vi "Histogram Main.vi"() -> ()   [LabVIEW 2012]
uses:
  Consumer Message.ctl
panel:
  out "波形图表":dbl[](graph)
  in  "快照":bool
  out "直方图":cluster{"histogram":dbl[], "x axis":dbl[]}(graph)
  out "消费者关闭？":bool
  in  "停止":bool
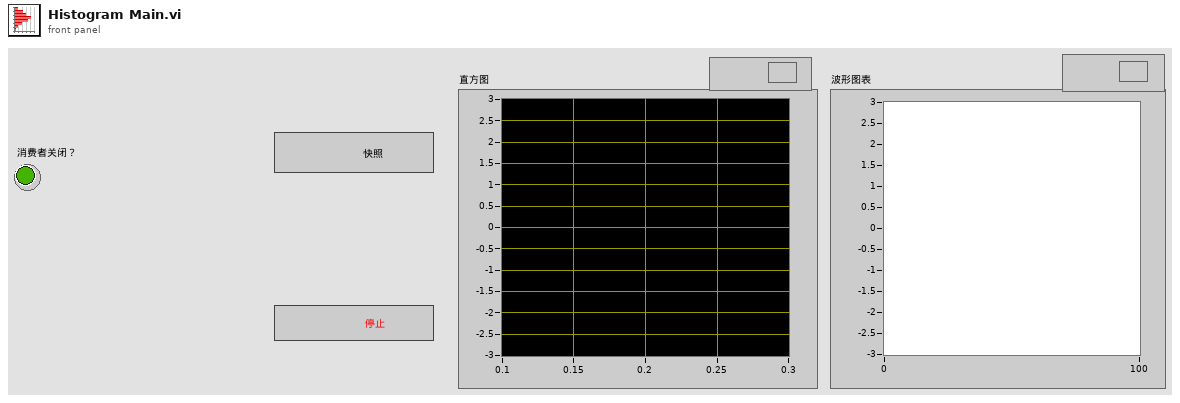
[diagram p1: front panel]
types:
  T1 = typedef "Consumer Message.ctl" = cluster{"消费者状态":string, "布尔数据":bool, "数值数据":i32, "信号":dbl[], "错误":cluster{"状态":bool, "代码":i32, "源":string}}
  T2 = enum32{"invalid app kind", "Development System", "Run Time System", "Student Edition", "Embedded LabVIEW", "Evaluation", "Custom"}
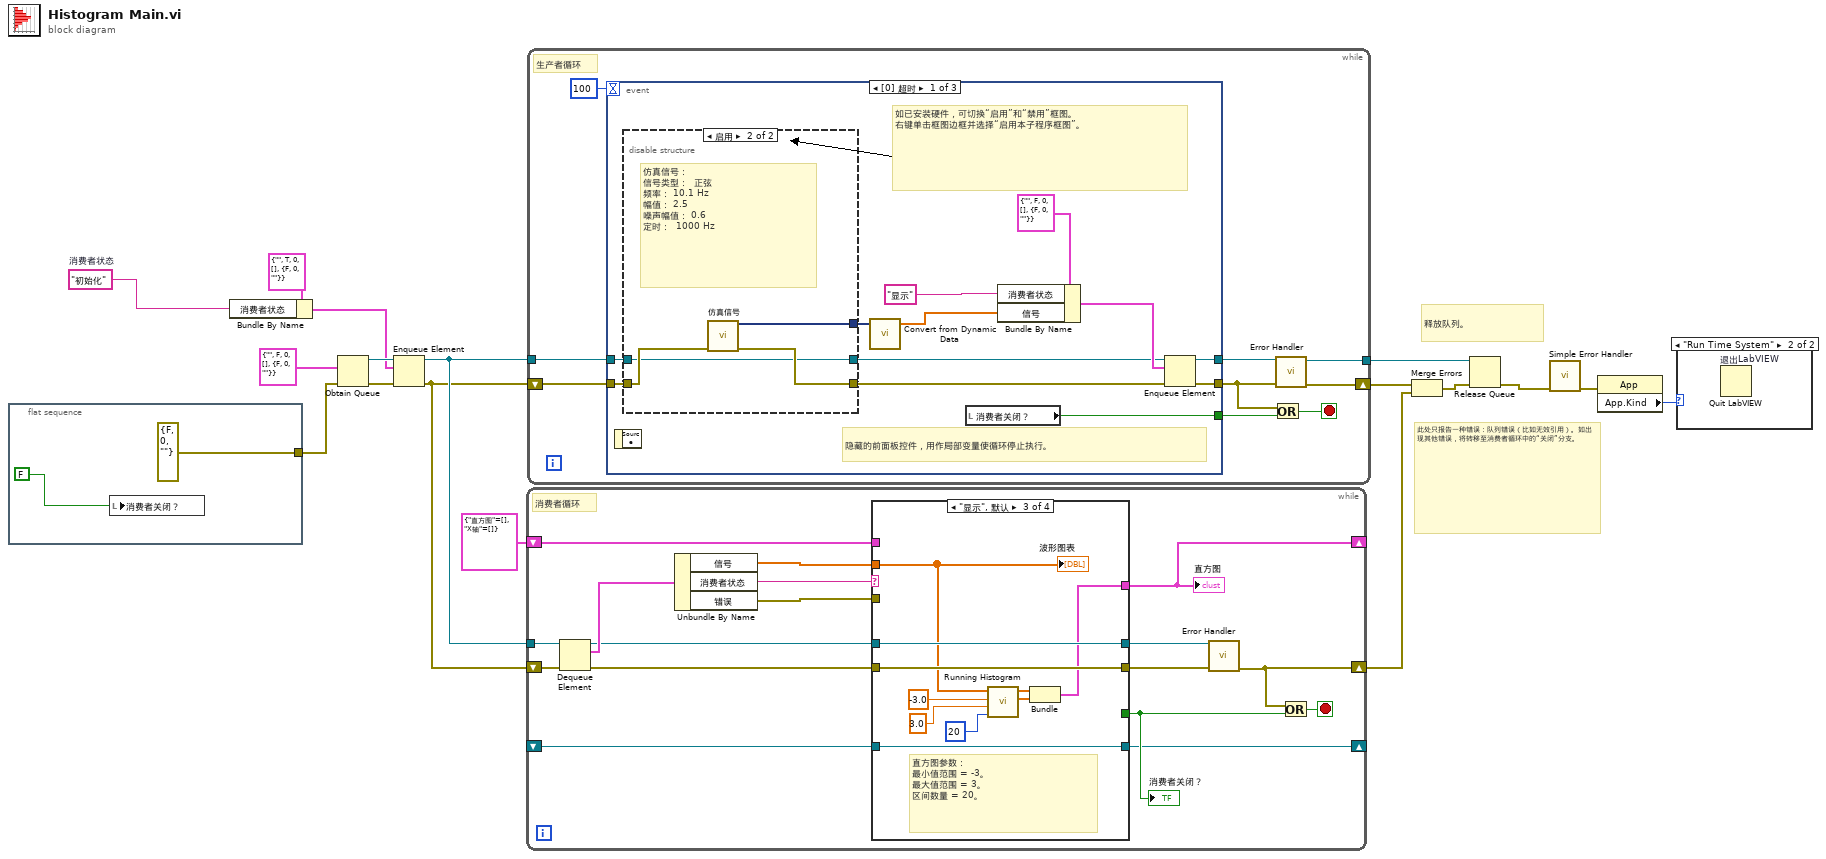
[diagram p0: block diagram]
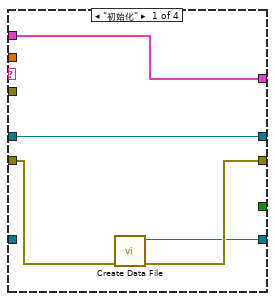
[diagram p3: hidden frame]
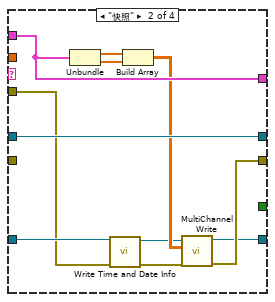
[diagram p4: hidden frame]
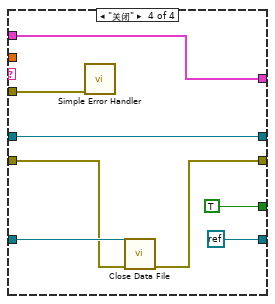
[diagram p5: hidden frame]
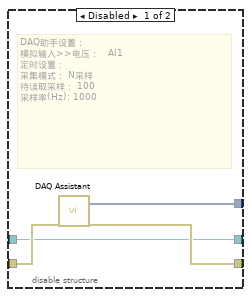
[diagram p6: hidden frame]
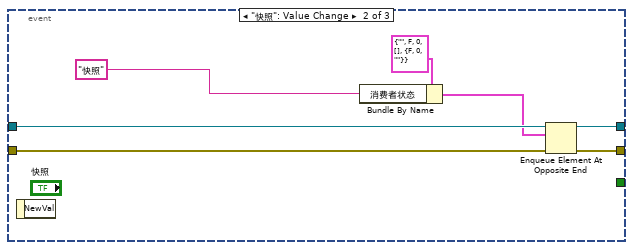
[diagram p7: hidden frame]
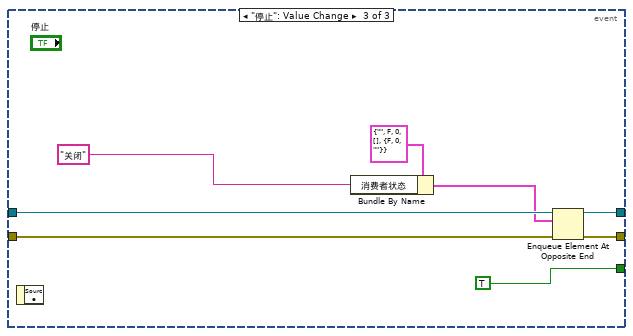
[diagram p8: hidden frame]
diagram:
  w10 = "初始化"  # 消费者状态
  # "释放队列。"
  # "此处只报告一种错误：队列错误（比如无效引用）。如出现其他错误，将转移至消费者循环中的“关闭”分支。"
  n1 = flat-sequence {
    tunnel: [cluster{"状态":bool, "代码":i32, "源":string} {"状态"=FALSE, "代码"=0, "源"=""} ("错误输入（无错误）")] -> w13
    frame #0 {
      n2 = local write "消费者关闭？"(FALSE ("停止循环（局部）")) -> ()
    }
  }
  n3 = Bundle By Name ("按名称捆绑")(cluster=T1 {"消费者状态"="", "布尔数据"=TRUE, "数值数据"=0, "信号"=[], "错误"={"状态"=FALSE, "代码"=0, "源"=""}} ("消费者消息"), "消费者状态"=w10) -> (w11:T1)
  n4 = Obtain Queue ("获取队列引用")(element data type=T1 {"消费者状态"="", "布尔数据"=FALSE, "数值数据"=0, "信号"=[], "错误"={"状态"=FALSE, "代码"=0, "源"=""}}, error in (no error)=w13) -> (queue out=w15:refnum<queue>, error out=w17:errorcluster)  [unwired: 3 in, 1 out]
  n5 = Enqueue Element ("元素入队列")(queue=w15, element=w11, error in (no error)=w17) -> (queue out=w14:refnum<queue>, error out=w4:errorcluster)  [unwired: 1 in, 1 out]
  n6 = while {
    tunnel: w14 -> [w36]
    shift-right: [w27] -> w8
    shift-left: w4 -> [w35]
    shift-right: [w20] -> _
    shift-left: cluster{"直方图":dbl[], "X轴":dbl[]} {"直方图"=[], "X轴"=[]} -> [w24]
    shift-right: [w21] -> _
    shift-left: _ -> [w22]
    stop <- w28 stop-if-true
    # "消费者循环"
    n7 = Dequeue Element ("元素出队列")(queue=w36, error in (no error)=w35) -> (queue out=w26:refnum<queue>, element=w34:T1, error out=w25:errorcluster)  [unwired: 1 in, 1 out]
    n8 = Unbundle By Name ("按名称解除捆绑")(w34) -> ("信号"=w23:dbl[], "消费者状态"=w33:string, "错误"=w30:cluster{"状态":bool, "代码":i32, "源":string})
    n9 = case shown="\"显示\", 默认" w33 {
      tunnel: [_ _ _ TRUE] -> w29
      tunnel: w25 -> [w39 _ w61 w65]
      tunnel: [w38 w48 w61 w64] -> w32
      tunnel: w26 -> [w41 w52 w62 w68]
      tunnel: [w41 w52 w62 w68] -> w31
      tunnel: w30 -> [_ w42 _ w69]
      tunnel: [w40 w50 w58 w67] -> w20
      tunnel: w24 -> [w40 w50 _ w67]
      tunnel: w23 -> [_ _ w56 _]
      tunnel: w22 -> [_ w43 w57 w66]
      tunnel: [w37 w47 w57 refnum<k0> refnum ("非法引用句柄常量")] -> w21
      frame "初始化" {
        n10 = call "Create Data File.vi"("错误输入"=w39) -> ("错误输出"=w38:cluster{"状态":bool, "代码":i32, "源":string}, "文件引用句柄"=w37:refnum<file>)  [unwired: 9 in]
      }
      frame "快照" {
        n11 = Unbundle ("解除捆绑")(w50) -> ("直方图"=w46:dbl[], "X轴"=w51:dbl[])
        n12 = call "Write Time and Date Info.vi"("错误输入"=w42, "文件引用句柄输入"=w43) -> ("错误输出"=w44:cluster{"状态":bool, "代码":i32, "源":string}, "文件引用句柄输出"=w45:refnum<file>)  [unwired: 6 in]
        n13 = Build Array ("创建数组")(w46, w51) -> (w49:dbl[][])
        n14 = call "MultiChannel Write.vi"("错误输入"=w44, "数据至记录"=w49, "文件引用句柄输入"=w45) -> ("错误输出"=w48:cluster{"状态":bool, "代码":i32, "源":string}, "文件引用句柄输出"=w47:refnum<file>)  [unwired: 7 in]
      }
      frame "显示", Default {
        # "直方图参数：\n最小值范围 = -3。\n最大值范围 = 3。\n区间数量 = 20。"
        n15 = call "Running Histogram.vi"("区间"=20, "最大值"=3.0, "最小值"=-3.0, "输入数据"=w56) -> ("X轴"=w59:dbl[], "直方图"=w60:dbl[])  [unwired: 4 in, 2 out]
        n16 = Bundle ("捆绑")("直方图"=w60, "X轴"=w59) -> (w58:cluster{"直方图":dbl[], "X轴":dbl[]})  [unwired: 1 in]
        "波形图表" <- w56
      }
      frame "关闭" {
        n17 = call <vilib>:"Simple Error Handler.vi"("error in (no error)"=w69) -> ()  [unwired: 4 in, 5 out]
        n18 = call "Close Data File.vi"("错误输入"=w65, "文件引用句柄输入"=w66) -> ("错误输出"=w64:errorcluster)  [unwired: 9 in]
      }
    }
    "消费者关闭？" <- w29
    "直方图" <- w20
    n19 = call "Error Handler.vi"("错误输入"=w32, "队列输入"=w31) -> ("错误输出"=w27:cluster{"状态":bool, "代码":i32, "源":string})  [unwired: 8 in, 1 out]
    n20 = Or ("或")(x=w27, y=w29) -> (x .or. y?=w28:bool)
  }
  n21 = while {
    tunnel: w14 -> [w79]
    shift-right: [w72] -> w9
    shift-left: w4 -> [w78]
    tunnel: [w71] -> w3
    stop <- w74 stop-if-true
    # "生产者循环"
    n22 = event shown="[0] 超时" {
      selector: _ -> [_ _ _]
      dyn-events: _ -> [_ _ _]
      timeout: 100 -> [_ _ _]
      tunnel: w79 -> [w81 w105 w114]
      tunnel: w78 -> [w83 w104 w112]
      tunnel: [w86 w106 w111] -> w73
      tunnel: [w91 _ TRUE] -> w75
      tunnel: [w87 w101 w110] -> w77
      event Timeout {
        # "如已安装硬件，可切换“启用”和“禁用”框图。\n右键单击框图边框并选择“启用本子程序框图”。"
        # "隐藏的前面板控件，用作局部变量使循环停止执行。"
        n23 = event-data ("事件数据节点")() -> ()  [unwired: 1 in, 1 out]
        n24 = disable-structure shown="启用" {
          disable-tunnel: [w95 w97] -> w84
          disable-tunnel: w83 -> [w94 w99]
          disable-tunnel: [w93 w98] -> w82
          disable-tunnel: w81 -> [w92 w96]
          disable-tunnel: [w92 w96] -> w80
          frame Disabled {
            # "DAQ助手设置：\n模拟输入>>电压：   AI1\n定时设置：\n采集模式： N采样\n待读取采样： 100\n采样率(Hz): 1000"
            n25 = call "DAQ Assistant"("error in"=w94) -> ("data"=w95:dynamicdata, "error out"=w93:errorcluster)  [unwired: 16 in, 1 out]
          }
          frame Enabled {
            # "仿真信号：\n信号类型：  正弦\n频率： 10.1 Hz\n幅值： 2.5\n噪声幅值： 0.6\n定时：  1000 Hz"
            n26 = call "仿真信号"("error in (no error)"=w99) -> ("正弦与均匀噪声"=w97:dynamicdata, "error out"=w98:errorcluster)  [unwired: 13 in]
          }
        }
        n27 = call "Convert from Dynamic Data"("Dynamic Data Type"=w84) -> ("Array"=w85:dbl[])  [unwired: 3 in]
        n28 = local read "消费者关闭？"() -> (w91:bool)
        n29 = Bundle By Name ("按名称捆绑")(cluster=T1 {"消费者状态"="", "布尔数据"=FALSE, "数值数据"=0, "信号"=[], "错误"={"状态"=FALSE, "代码"=0, "源"=""}}, "消费者状态"="显示", "信号"=w85) -> (w89:T1)
        n30 = Enqueue Element ("元素入队列")(queue=w80, element=w89, error in (no error)=w82) -> (queue out=w87:refnum<queue>, error out=w86:errorcluster)  [unwired: 1 in, 1 out]
      }
      event "快照": Value Change {
        n31 = event-data ("事件数据节点")() -> ()  [unwired: 1 in, 1 out]
        n32 = Bundle By Name ("按名称捆绑")(cluster=T1 {"消费者状态"="", "布尔数据"=FALSE, "数值数据"=0, "信号"=[], "错误"={"状态"=FALSE, "代码"=0, "源"=""}}, "消费者状态"="快照" ("字符串数据")) -> (w102:T1)
        n33 = Enqueue Element At Opposite End ("队列最前端插入元素")(queue=w105, element=w102, error in (no error)=w104) -> (queue out=w101:refnum<queue>, error out=w106:errorcluster)  [unwired: 1 in, 1 out]
      }
      event "停止": Value Change {
        n34 = event-data ("事件数据节点")() -> ()  [unwired: 1 in, 1 out]
        n35 = Bundle By Name ("按名称捆绑")(cluster=T1 {"消费者状态"="", "布尔数据"=FALSE, "数值数据"=0, "信号"=[], "错误"={"状态"=FALSE, "代码"=0, "源"=""}}, "消费者状态"="关闭") -> (w107:T1)
        n36 = Enqueue Element At Opposite End ("队列最前端插入元素")(queue=w114, element=w107, error in (no error)=w112) -> (queue out=w110:refnum<queue>, error out=w111:errorcluster)  [unwired: 1 in, 1 out]
      }
    }
    n37 = Or ("或")(x=w73, y=w75) -> (x .or. y?=w74:bool)
    n38 = call "Error Handler.vi"("错误输入"=w73, "队列输入"=w77) -> ("错误输出"=w72:cluster{"状态":bool, "代码":i32, "源":string}, "队列输出"=w71:refnum<queue>)  [unwired: 8 in]
  }
  n39 = Merge Errors ("合并错误")(w9, w8) -> (w6:errorcluster)
  n40 = Release Queue ("释放队列引用")(queue=w3, error in (no error)=w6) -> (error out=w5:errorcluster)  [unwired: 1 in, 2 out]
  n41 = call <vilib>:"Simple Error Handler.vi"("error in (no error)"=w5) -> ("error out"=w1:errorcluster)  [unwired: 4 in, 4 out]
  n42 = property on="属性节点" class="App"(error in=w1) -> ("App.Kind"=w2:T2)  [unwired: 1 in, 2 out]
  n43 = case shown="\"Run Time System\"" w2 {
    frame "invalid app kind", Default {
    }
    frame "Run Time System" {
      n44 = Quit LabVIEW "退出LabVIEW"() -> ()  [unwired: 1 in]
    }
  }
